vi "Main.vi"() -> ()   [LabVIEW 2020]
doc: "This template is for the Queued Message Handler design pattern.\n\nThe Event Handling Loop generates messages based on user interface actions.\n\nThe Message Handling Loop processes messages generated by the Event Handling Loop, or by other messages. The messages are string values, so new messages can be added easily to the Message Cases case structure in the Message Handling Loop. Each message cluster can also provide an optional value for Message Data, which is a variant that can be converted to whatever message-specific data is required."
uses:
  Pieces/Piece.lvclass
  Board/Board.lvclass
  <vilib>/Utility/error.llb/Error Cluster From Error Code.vi
  <vilib>/ErrorRing/Error Ring.xnode
  support/Message Queue/Message Queue.lvlib
  support/User Event - Stop/User Event - Stop.lvlib
panel:
  out "BoardDrawing":picture[][](array[picture])
  in  "Starting Position":string="rnbqkbnr/pppppppp/8/8/8/8/PPPPPPPP/RNBQKBNR w KQkq - 0 1"
  # "#ToDo\nPrint board design behind piece\nAdd legal moves highlight after piece is selected\nAdd piece movement\nAdd counters for movevements\nCheck castling rights\nAdd player turn alternation\nAdd capture\nAdd verification for check \nAdd verification for checkmate\nUndo movement\nAdd game control mechanics (start/restart/resign, etc.)\n\nFar far away goals:\nImplement StockFish engine interface"
  # "A"
  # "B"
  # "C"
  # "D"
  # "E"
  # "F"
  # "G"
  # "H"
  # "8"
  # "8"
  # "7"
  # "7"
  # "6"
  # "6"
  # "5"
  # "5"
  # "4"
  # "4"
  # "3"
  # "3"
  # "2"
  # "2"
  # "1"
  # "1"
  # "A"
  # "B"
  # "C"
  # "D"
  # "E"
  # "F"
  # "G"
  # "H"
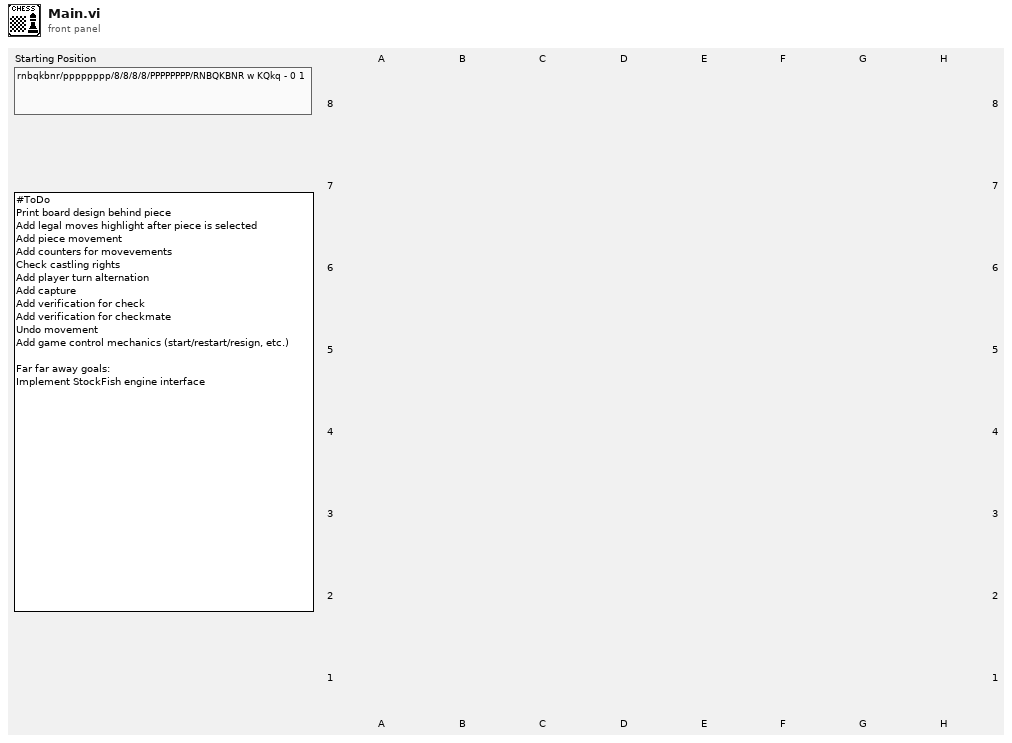
[diagram p1: front panel]
types:
  T1 = typedef "Message Queue.lvlib/All Message Queues.ctl" = cluster{"UI":refnum<queue>}
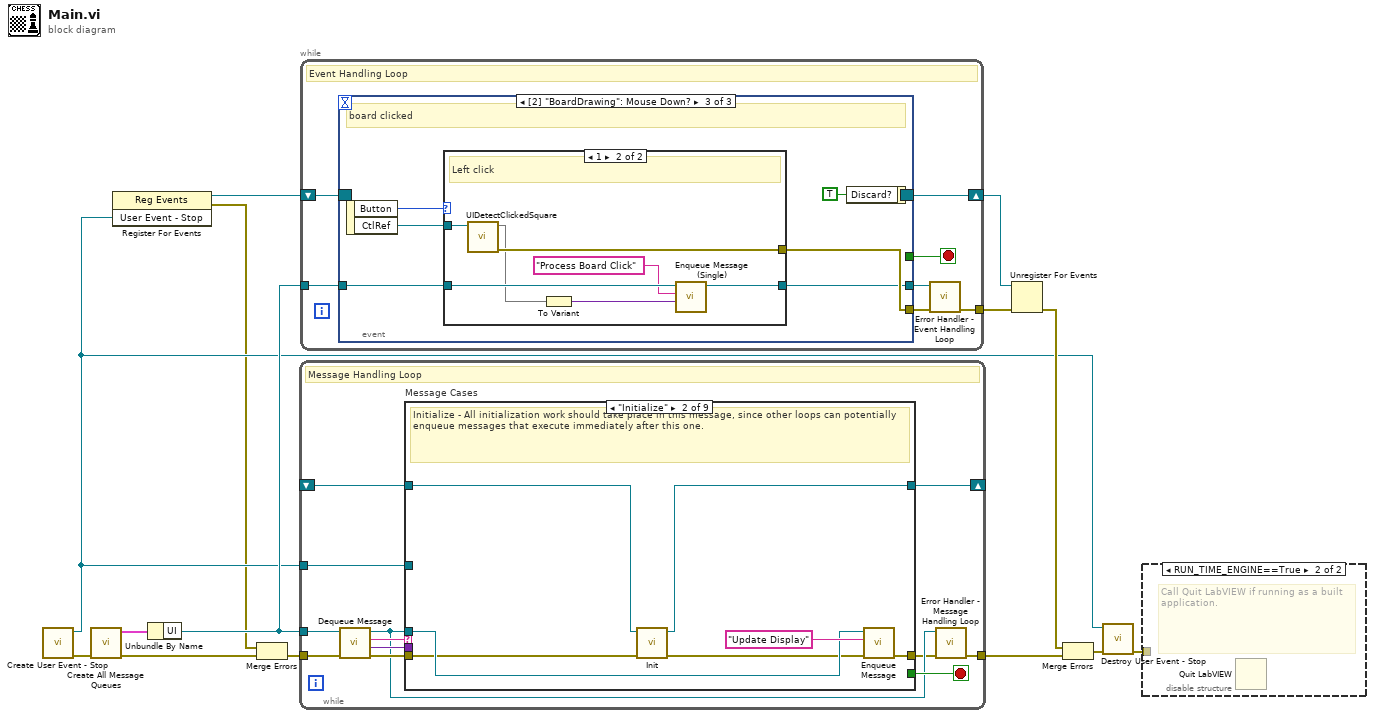
[diagram p0: block diagram]
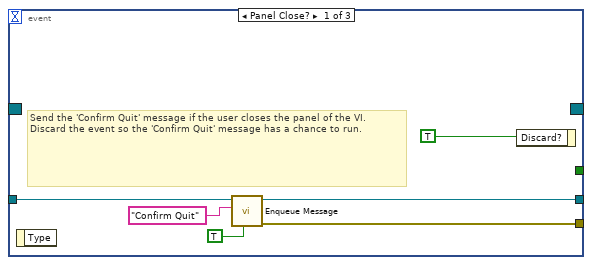
[diagram p3: hidden frame]
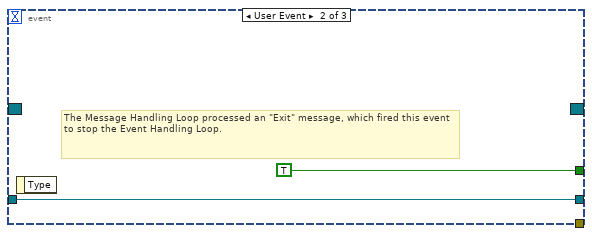
[diagram p4: hidden frame]
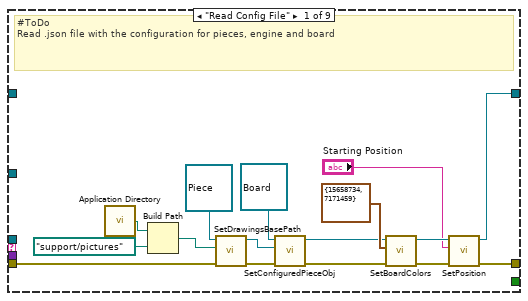
[diagram p6: hidden frame]
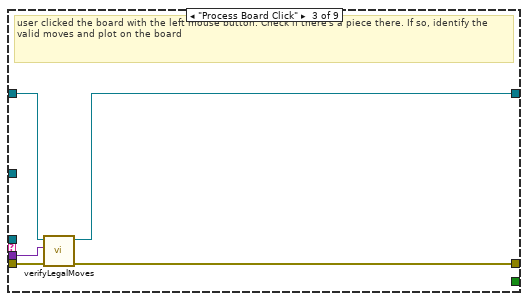
[diagram p7: hidden frame]
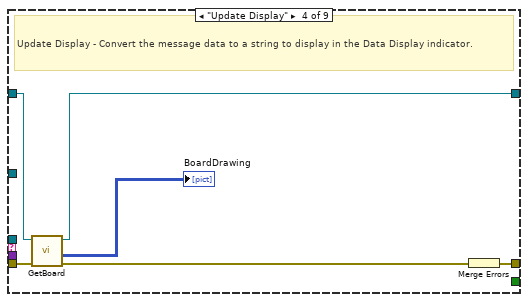
[diagram p8: hidden frame]
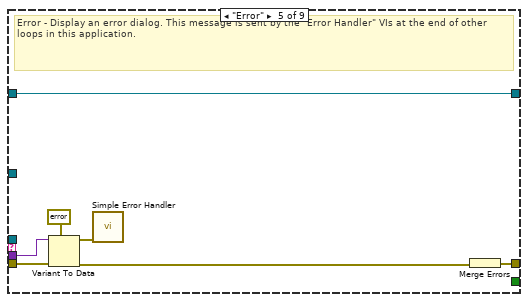
[diagram p9: hidden frame]
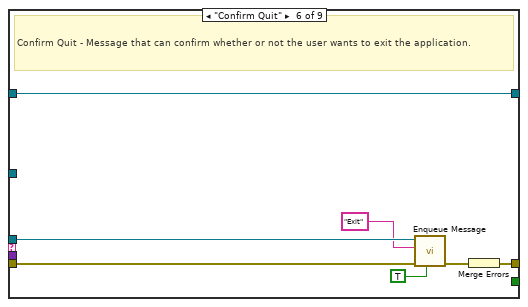
[diagram p10: hidden frame]
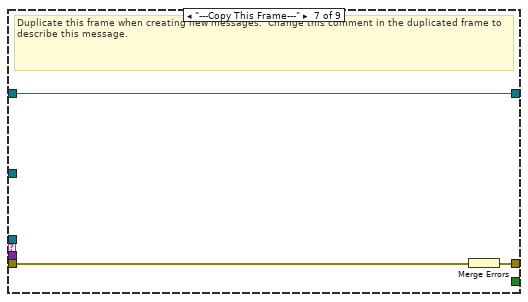
[diagram p11: hidden frame]
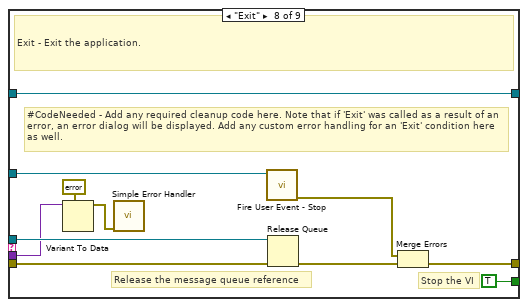
[diagram p12: hidden frame]
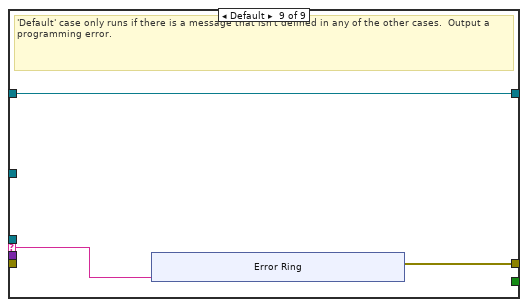
[diagram p13: hidden frame]
diagram:
  n1 = call "Create User Event - Stop.vi"() -> ("error out"=w10:errorcluster, "User Event - Stop"=w3:refnum<user-event>)  [unwired: 10 in]
  n2 = call "Create All Message Queues.vi"("error in (no error)"=w10) -> ("error out"=w14:errorcluster, "Message Queues out"=w13:T1)  [unwired: 9 in]
  n3 = register-events(w3) -> (reference out=w4:refnum<event-registration>, error out=w1:errorcluster)  [unwired: 2 in]
  n4 = Unbundle By Name(w13) -> ("UI"=w11:refnum<queue>)
  n5 = Merge Errors(w1, w14) -> (w2:errorcluster)
  n6 = while {
    tunnel: w11 -> [w18]
    shift-right: [w25] -> _
    shift-left: _ -> [w26]
    tunnel: w3 -> [w23]
    tunnel: w2 -> [w22]
    tunnel: [w16] -> w12
    stop <- w24 stop-if-true
    # "Message Handling Loop"
    n7 = call "Dequeue Message.vi"("error in (no error)"=w22, "Message Queue"=w18) -> ("error out"=w21:errorcluster, "Message Data"=w19:variant, "Message"=w20:string, "dup Message Queue"=w17:refnum<queue>)  [unwired: 6 in]
    n8 = case "Message Cases" shown="\"Initialize\"" w20 {
      selector: w20 -> [_ _ _ _ _ _ _ _ w89]
      tunnel: w17 -> [_ w47 _ _ _ w70 _ w88 _]
      tunnel: w21 -> [w36 w44 w54 w59 w67 w74 w77 w81 _]
      tunnel: [w30 w49 w53 w60 w61 w72 w75 w84 w90] -> w15
      tunnel: w26 -> [_ w46 w52 w57 w66 w73 w76 w87 w91]
      tunnel: [w28 w45 w51 w56 w66 w73 w76 w87 w91] -> w25
      tunnel: [_ _ _ _ _ _ _ TRUE _] -> w24
      tunnel: w19 -> [_ _ w50 _ w65 _ _ w78 _]
      tunnel: w23 -> [_ _ _ _ _ _ _ w83 _]
      frame "Read Config File" {
        # "#ToDo\nRead .json file with the configuration for pieces, engine and board"
        n9 = call <vilib>:"Application Directory.vi"() -> ("Application Directory"=w39:path)
        n10 = Build Path(base path=w39, name or relative path=path "support/pictures") -> (appended path=w40:path)
        n11 = call "SetDrawingsBasePath.vi"("error in (no error)"=w36, "drawingsBasePath"=w40, "object in"=refnum<class "Piece.lvclass"> refnum) -> ("error out"=w35:errorcluster, "object out"=w31:refnum<class "Piece.lvclass">)  [unwired: 7 in]
        n12 = call "SetConfiguredPieceObj.vi"("error in (no error)"=w35, "configuredPieceObj"=w31, "object in"=refnum<class "Board.lvclass"> refnum) -> ("error out"=w34:errorcluster, "object out"=w32:refnum<class "Board.lvclass">)  [unwired: 7 in]
        n13 = call "SetBoardColors.vi"("error in (no error)"=w34, "boardColors"=cluster{"light":u32, "dark":u32} {"light"=15658734, "dark"=7171459}, "object in"=w32) -> ("error out"=w42:errorcluster, "object out"=w29:refnum<class "Board.lvclass">)  [unwired: 7 in]
        n14 = call "SetPosition.vi"("error in (no error)"=w42, "position (\"\")"="Starting Position", "object in"=w29) -> ("error out"=w30:errorcluster, "object out"=w28:refnum<class "Board.lvclass">)  [unwired: 7 in]
      }
      frame "Initialize" {
        # "Initialize - All initialization work should take place in this message, since other loops can potentially enqueue messages that execute immediately after this one."
        n15 = call "Init.vi"("error in (no error)"=w44, "object in"=w46) -> ("error out"=w43:errorcluster, "object out"=w45:refnum<class "Board.lvclass">)  [unwired: 8 in]
        n16 = call-poly "Enqueue Message.vi"("error in (no error)"=w43, "Message"="Update Display", "Message Queue"=w47) -> ("error out"=w49:errorcluster)  [unwired: 7 in, 1 out]
      }
      frame "Process Board Click" {
        # "user clicked the board with the left mouse button. Check if there's a piece there. If so, identify the valid moves and plot on the board"
        n17 = call-dynamic "verifyLegalMoves.vi"("error in (no error)"=w54, "Index"=w50, "object in"=w52) -> ("error out"=w53:errorcluster, "object out"=w51:refnum<class "Board.lvclass">)  [unwired: 7 in]
      }
      frame "Update Display" {
        # "Update Display - Convert the message data to a string to display in the Data Display indicator."
        n18 = call "GetBoard.vi"("error in (no error)"=w59, "object in"=w57) -> ("error out"=w58:errorcluster, "BoardDrawing"=→"BoardDrawing":picture[][], "object out"=w56:refnum<class "Board.lvclass">)  [unwired: 6 in, 1 out]
        n19 = Merge Errors(w58) -> (w60:errorcluster)
      }
      frame "Error" {
        # "Error - Display an error dialog. This message is sent by the \"Error Handler\" VIs at the end of other loops in this application."
        n20 = Variant To Data(error in=w67, type=errorcluster {"status"=FALSE, "code"=0, "source"=""} ("error constant"), Variant=w65) -> (data=w63:errorcluster, error out=w62:errorcluster)
        n21 = call <vilib>:"Simple Error Handler.vi"("error in (no error)"=w63) -> ()  [unwired: 4 in, 5 out]
        n22 = Merge Errors(w62) -> (w61:errorcluster)
      }
      frame "Confirm Quit" {
        # "Confirm Quit - Message that can confirm whether or not the user wants to exit the application."
        n23 = call-poly "Enqueue Message.vi"("Priority Message? (F)"=TRUE, "error in (no error)"=w74, "Message"="Exit", "Message Queue"=w70) -> ("error out"=w71:errorcluster)  [unwired: 6 in, 1 out]
        n24 = Merge Errors(w71) -> (w72:errorcluster)
      }
      frame "---Copy This Frame---" {
        # "Duplicate this frame when creating new messages.  Change this comment in the duplicated frame to describe this message."
        n25 = Merge Errors(w77) -> (w75:errorcluster)
      }
      frame "Exit" {
        # "Stop the VI"
        # "Release the message queue reference"
        # "#CodeNeeded - Add any required cleanup code here. Note that if 'Exit' was called as a result of an error, an error dialog will be displayed. Add any custom error handling for an 'Exit' condition here as well."
        # "Exit - Exit the application."
        n26 = Variant To Data(type=errorcluster {"status"=FALSE, "code"=0, "source"=""} ("error constant"), Variant=w78) -> (data=w79:errorcluster)  [unwired: 1 in, 1 out]
        n27 = call <vilib>:"Simple Error Handler.vi"("error in (no error)"=w79) -> ()  [unwired: 4 in, 5 out]
        n28 = call "Fire User Event - Stop.vi"("User Event - Stop"=w83) -> ("error out"=w82:errorcluster)  [unwired: 10 in]
        n29 = Release Queue(queue=w88, error in (no error)=w81) -> (error out=w85:errorcluster)  [unwired: 1 in, 2 out]
        n30 = Merge Errors(w82, w85) -> (w84:errorcluster)
      }
      frame Default {
        # "'Default' case only runs if there is a message that isn't defined in any of the other cases.  Output a programming error."
        n31 = xnode "Error Ring"("parameter 0"=w89) -> ("error out"=w90:errorcluster)
      }
    }
    n32 = call "Error Handler - Message Handling Loop.vi"("error in (no error)"=w15, "Message Queue"=w17) -> ("dup error in"=w16:errorcluster)  [unwired: 8 in, 1 out]
  }
  n33 = while {
    tunnel: w11 -> [w105]
    shift-right: [w103] -> w7
    shift-left: w4 -> [w104]
    tunnel: [w99] -> w5
    stop <- w101 stop-if-true
    # "Event Handling Loop"
    n34 = event shown="[2] \"BoardDrawing\": Mouse Down?" {
      selector: w104 -> [_ _ _]
      dyn-events: [_ _ _] -> w103
      timeout: _ -> [_ _ _]
      tunnel: [_ TRUE ("Discard?") _] -> w101
      tunnel: w105 -> [w110 w113 w119]
      tunnel: [w109 _ w117] -> w102
      tunnel: [w108 w113 w116] -> w100
      event Panel Close? {
        # "Send the 'Confirm Quit' message if the user closes the panel of the VI. Discard the event so the 'Confirm Quit' message has a chance to run."
        n35 = event-data() -> ()  [unwired: 1 in, 1 out]
        n36 = call-poly "Enqueue Message.vi"("Priority Message? (F)"=TRUE, "Message"="Confirm Quit", "Message Queue"=w110) -> ("error out"=w109:errorcluster, "dup Message Queue"=w108:refnum<queue>)  [unwired: 7 in]
        n37 = event-data("Discard?"=TRUE) -> ()  [unwired: 1 in, 1 out]
      }
      event User Event {
        # "The Message Handling Loop processed an \"Exit\" message, which fired this event to stop the Event Handling Loop."
        n38 = event-data() -> ()  [unwired: 1 in, 1 out]
      }
      event "BoardDrawing": Mouse Down? {
        # "board clicked"
        n39 = event-data() -> ("Button"=w114:u16, "CtlRef"=w118:refnum<vi>)  [unwired: 1 in]
        n40 = case shown="1" w114 {
          tunnel: w119 -> [w120 w127]
          tunnel: w118 -> [_ w126]
          tunnel: [_ w125] -> w117
          tunnel: [w120 w124] -> w116
          frame 0, Default {
            # "right click or something else"
          }
          frame 1 {
            # "Left click"
            n41 = call "UIDetectClickedSquare.vi"("Array in"=w126) -> ("error out"=w125:errorcluster, "Map"=w121:map{string, i32})  [unwired: 9 in]
            n42 = To Variant(anything=w121) -> (Variant=w123:variant)
            n43 = call "Enqueue Message (Single).vi"("Message Data"=w123, "Message"="Process Board Click", "Message Queue"=w127) -> ("dup Message Queue"=w124:refnum<queue>)  [unwired: 7 in, 1 out]
          }
        }
        n44 = event-data("Discard?"=TRUE) -> ()  [unwired: 1 in, 1 out]
      }
    }
    n45 = call "Error Handler - Event Handling Loop.vi"("error in (no error)"=w102, "Message Queue"=w100) -> ("dup error in"=w99:errorcluster)  [unwired: 8 in, 1 out]
  }
  n46 = Unregister For Events(event registration refnum=w7, error in=w5) -> (error out=w8:errorcluster)
  n47 = Merge Errors(w8, w12) -> (w9:errorcluster)
  n48 = call "Destroy User Event - Stop.vi"("error in (no error)"=w9, "User Event - Stop"=w3) -> ("error out"=w6:errorcluster)  [unwired: 9 in]
  n49 = disable-structure shown="RUN_TIME_ENGINE==True" {
    disable-tunnel: w6 -> [_ _]
    frame condition #0 (active) {
    }
    frame condition #1 {
      # "Call Quit LabVIEW if running as a built application."
      n50 = Quit LabVIEW() -> ()  [unwired: 1 in]
    }
  }
